vi "Dispense FN - ON - Measure Slope (SubVI).vi"(0 "Measured Mass (g)":dbl(knob) scale=0.0..100.0, 1 "Slope Sample Time (s)":dbl=0.5, 2 "Slope Limits (± g/sec)":dbl=10.0, 3 "Slope Level Range (± g/sec)":dbl=0.25, 4 "Slope Ave Array Size":i32=5, 5 "Initialize":bool) -> (14 "Level Signal":bool, 15 "Ave. Slope (g/sec)":dbl, 16 "Rate (g/sec)":dbl, 17 "Time (s)":dbl)   [LabVIEW 2012]
uses:
  <vilib>/ptbypt/NI_PtbyPt.lvlib
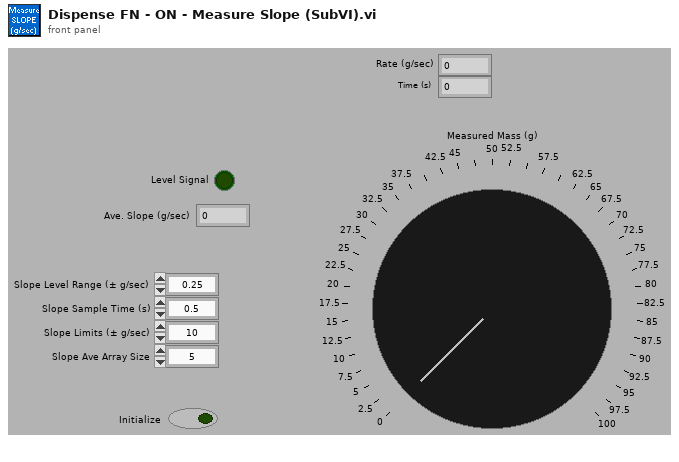
[diagram p1: front panel]
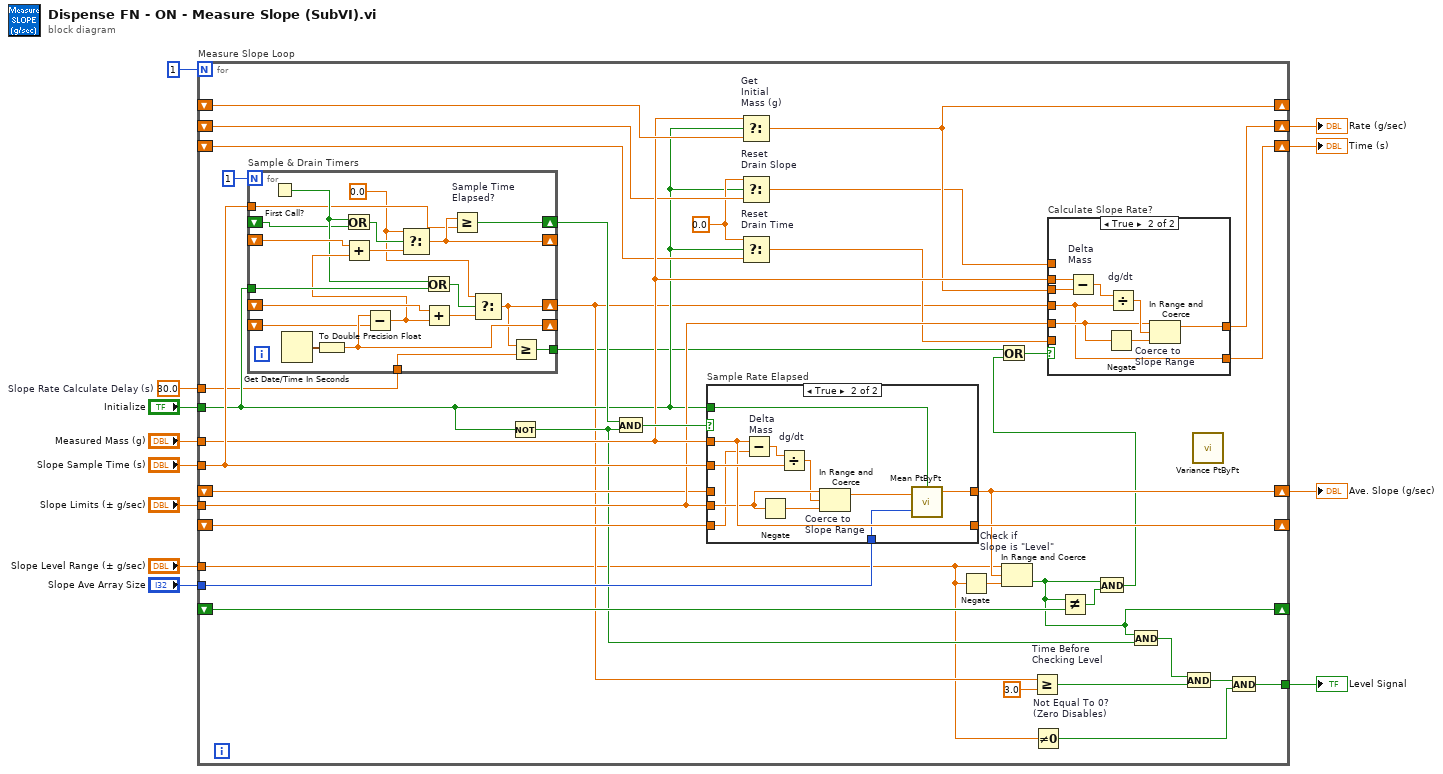
[diagram p0: block diagram]
diagram:
  w1 = 30.0  # Slope Rate Calculate Delay (s)
  n1 = for "Measure Slope Loop" {
    N: 1 -> [_]
    tunnel: "Measured Mass (g)" -> [w43]
    shift-right: [w50] -> _
    shift-left: _ -> [w28]
    shift-right: [w30] -> w7
    shift-left: _ -> [w27]
    tunnel: "Slope Sample Time (s)" -> [w46]
    tunnel: "Initialize" -> [w29]
    tunnel: "Slope Limits (± g/sec)" -> [w41]
    tunnel: "Slope Level Range (± g/sec)" -> [w20]
    tunnel: "Slope Ave Array Size" -> [w48]
    shift-right: [w42] -> _
    shift-left: _ -> [w44]
    shift-right: [w26] -> _
    shift-left: _ -> [w39]
    shift-right: [w40] -> w4
    shift-left: _ -> [w37]
    shift-right: [w35] -> w3
    shift-left: _ -> [w34]
    tunnel: [w17] -> w2
    tunnel: w1 -> [w16]
    w33 = 0.0 ("t")
    n2 = for "Sample & Drain Timers" {
      N: 1 -> [_]
      shift-right: [w62] -> w24
      shift-left: _ -> [w80]
      shift-right: [w76] -> _
      shift-left: _ -> [w75]
      tunnel: w29 -> [w74]
      shift-right: [w70] -> _
      shift-left: _ -> [w69]
      tunnel: w46 -> [w67]
      shift-right: [w66] -> w45
      shift-left: _ -> [w64]
      tunnel: w16 -> [w63]
      tunnel: [w61] -> w15
      w65 = 0.0 ("t")
      n3 = First Call?() -> (First Call?: T/F=w68:bool)
      n4 = Get Date/Time In Seconds() -> (seconds since 1Jan1904=w79:timestamp)
      n5 = To Double Precision Float(number=w79) -> (double precision float=w76:dbl)
      n6 = Or(x=w68, y=w64) -> (x .or. y?=w72:bool)
      n7 = Subtract(x=w76, y=w75) -> (x-y=w71:dbl)
      n8 = Add(x=w69, y=w71) -> (x+y=w73:dbl)
      n9 = Select(t=w65, s=w72, f=w73) -> (s? t:f=w70:dbl)
      n10 = Or(x=w68, y=w74) -> (x .or. y?=w77:bool)
      n11 = Add(x=w80, y=w71) -> (x+y=w78:dbl)
      n12 = Greater Or Equal? "Sample Time\nElapsed?"(x=w70, y=w67) -> (x >= y?=w66:bool)
      n13 = Select(t=w65, s=w77, f=w78) -> (s? t:f=w62:dbl)
      n14 = Greater Or Equal?(x=w62, y=w63) -> (x >= y?=w61:bool)
    }
    n15 = Not(x=w29) -> (.not. x?=w25:bool)
    n16 = And(x=w45, y=w25) -> (x .and. y?=w49:bool)
    n17 = case "Sample Rate Elapsed" shown="True" w49 {
      tunnel: w43 -> [_ w91]
      tunnel: [w82 w84] -> w30
      tunnel: [w81 w91] -> w50
      tunnel: w46 -> [_ w92]
      tunnel: w41 -> [_ w90]
      tunnel: w48 -> [_ w88]
      tunnel: w29 -> [_ w87]
      tunnel: w28 -> [w81 w86]
      tunnel: w27 -> [w82 _]
      frame False {
      }
      frame True {
        n18 = Subtract "Delta\nMass"(x=w91, y=w86) -> (x-y=w93:dbl)
        n19 = Negate(x=w90) -> (-x=w89:dbl)
        n20 = Divide "dg/dt"(x=w93, y=w92) -> (x/y=w83:dbl)
        n21 = In Range and Coerce "Coerce to\nSlope Range"(upper limit=w90, x=w83, lower limit=w89) -> (coerced(x)=w85:dbl)  [unwired: 1 out]
        n22 = call <vilib>:"Mean PtByPt.vi"("x"=w85, "sample length"=w88, "initialize"=w87) -> ("mean"=w84:dbl)  [unwired: 2 out]
      }
    }
    n23 = Select "Get\nInitial\nMass (g)"(t=w43, s=w29, f=w44) -> (s? t:f=w42:dbl)
    n24 = Select "Reset\nDrain Slope"(t=w33, s=w29, f=w37) -> (s? t:f=w36:dbl)
    n25 = Select "Reset\nDrain Time"(t=w33, s=w29, f=w34) -> (s? t:f=w32:dbl)
    n26 = Negate(x=w20) -> (-x=w31:dbl)
    n27 = In Range and Coerce "Check if\nSlope is \"Level\""(upper limit=w20, x=w30, lower limit=w31) -> (In Range?=w26:bool)  [unwired: 1 out]
    n28 = Greater Or Equal? "Time Before\nChecking Level"(x=w24, y=3.0) -> (x >= y?=w22:bool)
    n29 = Not Equal To 0? "Not Equal To 0?\n(Zero Disables)"(x=w20) -> (x != 0?=w18:bool)
    n30 = Not Equal?(x=w26, y=w39) -> (x != y?=w38:bool)
    n31 = And(x=w26, y=w38) -> (x .and. y?=w14:bool)
    n32 = Or(x=w15, y=w14) -> (x .or. y?=w13:bool)
    n33 = case "Calculate Slope Rate?" shown="True" w13 {
      tunnel: w43 -> [_ w58]
      tunnel: w42 -> [_ w54]
      tunnel: w24 -> [_ w53]
      tunnel: w41 -> [_ w56]
      tunnel: [w52 w55] -> w40
      tunnel: w36 -> [w52 _]
      tunnel: [w51 w53] -> w35
      tunnel: w32 -> [w51 _]
      frame False {
      }
      frame True {
        n34 = Subtract "Delta\nMass"(x=w58, y=w54) -> (x-y=w57:dbl)
        n35 = Negate(x=w56) -> (-x=w60:dbl)
        n36 = Divide "dg/dt"(x=w57, y=w53) -> (x/y=w59:dbl)
        n37 = In Range and Coerce "Coerce to\nSlope Range"(upper limit=w56, x=w59, lower limit=w60) -> (coerced(x)=w55:dbl)  [unwired: 1 out]
      }
    }
    n38 = And(x=w26, y=w25) -> (x .and. y?=w21:bool)
    n39 = And(x=w21, y=w22) -> (x .and. y?=w19:bool)
    n40 = call <vilib>:"Variance PtByPt.vi"() -> ()  [unwired: 3 in, 3 out]
    n41 = And(x=w19, y=w18) -> (x .and. y?=w17:bool)
  }
  "Ave. Slope (g/sec)" <- w7
  "Level Signal" <- w2
  "Rate (g/sec)" <- w4
  "Time (s)" <- w3
